vi "dynamatic.vi"(8 "error in (no error)":errorcluster, 11 "IBar in":refnum<class "IBar.lvclass">) -> (0 "error out":errorcluster, 2 "String":string, 3 "IBar out":refnum<class "IBar.lvclass">)   [LabVIEW 2021, in "IBar.lvclass"]
uses:
  IBar.lvclass
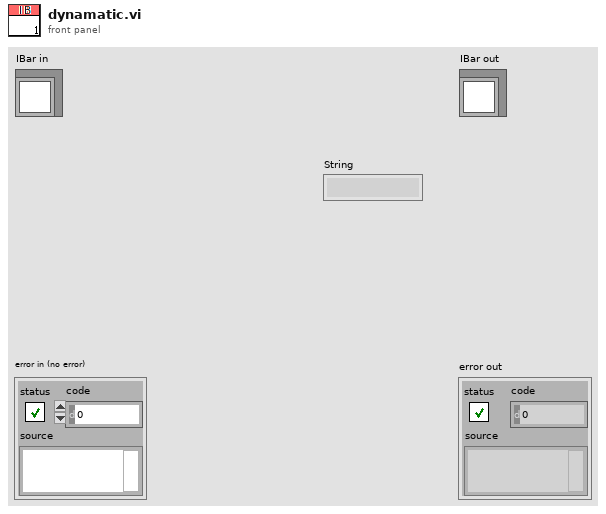
[diagram p1: front panel]
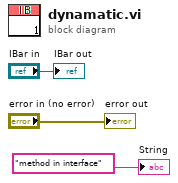
[diagram p0: block diagram]
diagram:
  "error out" <- "error in (no error)"
  "IBar out" <- "IBar in"
  "String" <- "method in interface"
